vi "Read State.vi"(8 "error in (no error)":errorcluster, 11 "signal configuration":refnum<class "SV Signal.lvclass">) -> (0 "error out":errorcluster, 2 "generator state":T3={"system timing model"=10178, "state"={"RESET"=FALSE, "generator timestamp"=timestamp(0 s since 1904-01-01), "elapsed seconds"=0.0, "elapsed samples"=0, "generation state"=enum."Idle", "time offset at state"=0.0, "samples generated at state"=0, "signal state"=variant}, "duration of state"=0.0, "samples remaining at state"=0} {"system timing model" items=["Finite"=10178, "-"=-1, "Continuous"=10123, "-"=-2, "Settled"=110123, "Averaged"=210123, "Discrete Sweep"=310123, "Continuous Sweep"=410123]}, 3 "signal configuration":refnum<class "SV Signal.lvclass">)   [LabVIEW 2017, in "SV Signal.lvclass"]
uses:
  <vilib>/addons/_NISVFA/_Generation/Signal Generation/SV Signal/SV Signal.lvclass
  <vilib>/addons/_NISVFA/_Generation/Signal Generation/SV Signal/sv_System Timing Model.ctl
  <vilib>/addons/_NISVFA/_Generation/Signal Generation/SV Signal/sv_Generation State.ctl
  <vilib>/addons/_NISVFA/_Generation/Signal Generation/SV Signal/SV Signal.lvclass/SV Signal.ctl
  <vilib>/addons/_NISVFA/_Generation/SoundVib_Generation.lvlib
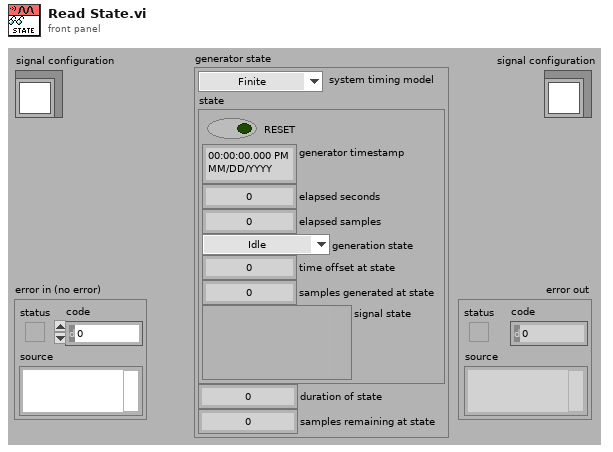
[diagram p1: front panel]
types:
  T1 = typedef "SV Signal.lvclass/sv_System Timing Model.ctl" = i64
  T2 = typedef "SV Signal.lvclass/sv_Generation State.ctl" = enum16{"Idle", "Ramp Up", "Pre-Measurement Settling", "Measurement", "Post-Measurement Settling", "Discrete Sweep Transition", "Ramp Down", "Update"}
  T3 = cluster{"system timing model":T1, "state":cluster{"RESET":bool, "generator timestamp":timestamp, "elapsed seconds":dbl, "elapsed samples":u64, "generation state":T2, "time offset at state":dbl, "samples generated at state":u64, "signal state":variant}, "duration of state":dbl, "samples remaining at state":i32}
  T4 = cluster{"RESET":bool, "generator timestamp":timestamp, "elapsed seconds":dbl, "elapsed samples":u64, "generation state":T2, "time offset at state":dbl, "samples generated at state":u64, "signal state":variant}
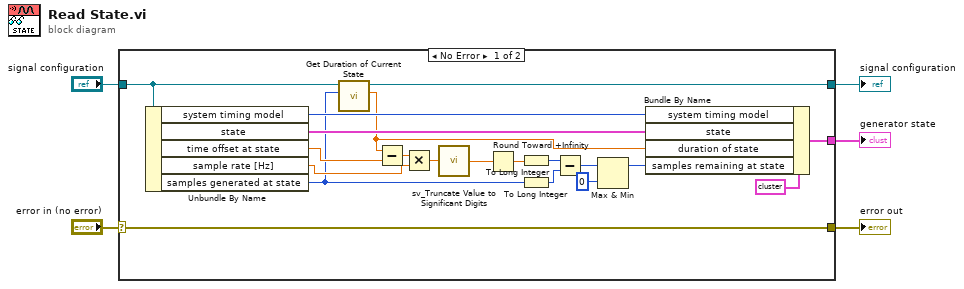
[diagram p0: block diagram]
diagram:
  n1 = case shown="No Error" "error in (no error)" {
    selector: "error in (no error)" -> [w25 w26]
    tunnel: [w25 w26] -> w4
    tunnel: [w20 w27] -> w2
    tunnel: "signal configuration" -> [w19 w27]
    tunnel: [w22 _] -> w1
    frame No Error {
      n2 = Unbundle By Name(w19) -> ("system timing model"=w23:T1, "state"=w18:T4, "time offset at state"=w17:dbl, "sample rate [Hz]"=w21:dbl, "samples generated at state"=w6:u64)
      n3 = call-dynamic "Get Duration of Current State.vi"("samples generated at state"=w6, "signal configuration"=w19) -> ("current state duration [s]"=w16:dbl, "signal configuration"=w20:refnum<class "SV Signal.lvclass">)  [unwired: 8 in]
      n4 = Subtract(x=w16, y=w17) -> (x-y=w24:dbl)
      n5 = Multiply(x=w24, y=w21) -> (x*y=w9:dbl)
      n6 = call <vilib>:"sv_Truncate Value to Significant Digits.vi"("value"=w9) -> ("truncated value"=w8:dbl)  [unwired: 14 in]
      n7 = Round Toward +Infinity(x=w8) -> (ceil(x): smallest int >= x=w7:dbl)
      n8 = To Long Integer(number=w7) -> (32bit integer=w13:i32)
      n9 = To Long Integer(number=w6) -> (32bit integer=w11:i32)
      n10 = Subtract(x=w13, y=w11) -> (x-y=w12:i32)
      n11 = Max & Min(x=w12, y=0) -> (max(x,y)=w10:i32)  [unwired: 1 out]
      n12 = Bundle By Name(cluster=T3 {"system timing model"=10178, "state"={"RESET"=FALSE, "generator timestamp"=timestamp(0 s since 1904-01-01), "elapsed seconds"=0.0, "elapsed samples"=0, "generation state"=enum."Idle", "time offset at state"=0.0, "samples generated at state"=0, "signal state"=variant}, "duration of state"=0.0, "samples remaining at state"=0} ("generator state"), "system timing model"=w23, "state"=w18, "duration of state"=w16, "samples remaining at state"=w10) -> (w22:T3)
    }
    frame Error {
    }
  }
  "error out" <- w4
  "signal configuration" <- w2
  "generator state" <- w1
